vi "Drive_Execute.vi"() -> ()   [LabVIEW 2019]
uses:
  Drive_Globals.vi
  <vilib>/Rock Robotics/WPI/ThirdParty/Phoenix-LabVIEW/Motor Controller/Controls/CTRE_Phoenix_MotorControl_ControlMode.ctl
  <vilib>/Rock Robotics/WPI/Joystick/WPI_JoystickArcadeMapping.vi
panel:
  in  "Max Speed":dbl
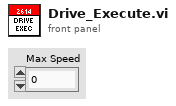
[diagram p1: front panel]
types:
  T1 = typedef "WPI_MotorControlDeviceRef.ctl" = cluster{"DeviceStatus":errorcluster, "Type":T2, "PWM":cluster{"PWM Channel":T3, "DeadBand":T4}, "CAN":cluster{"Device Number":u8, "SetOutput VI Ref":variant, "GetOutput VI Ref":variant, "Enable VI Ref":variant, "Disable VI Ref":variant, "Data":variant}, "Invert":bool, "DIO PWM":cluster{"PWM \"Enable\" Channel":T3, "DIOChannel":T5, "PWM Rate":dbl}}
  T2 = typedef "WPI_MotorControlType.ctl" = enum16{"PWM", "CAN", "DIO PWM"}
  T3 = typedef "FPGA_DIOPWMChannel.ctl" = enum8{"PWM 0", "PWM 1", "PWM 2", "PWM 3", "PWM 4", "PWM 5", "PWM 6", "PWM 7", "PWM 8", "PWM 9", "PWM MXP 0", "PWM MXP 1", "PWM MXP 2", "PWM MXP 3", "PWM MXP 4", "PWM MXP 5", "PWM MXP 6", "PWM MXP 7", "PWM MXP 8", "PWM MXP 9", "Invalid"}
  T4 = typedef "WPI_PWMDeadband.ctl" = cluster{"Name":string, "maxPositivePwm":i32, "minPositivePwm":i32, "centerPwm":i32, "maxNegativePwm":i32, "minNegativePwm":i32, "angularRange":u16}
  T5 = typedef "FPGA_DIOChannel.ctl" = enum8{"DIO 0", "DIO 1", "DIO 2", "DIO 3", "DIO 4", "DIO 5", "DIO 6", "DIO 7", "DIO 8", "DIO 9", "DIO MXP 0", "DIO MXP 1", "DIO MXP 2", "DIO MXP 3", "DIO MXP 4", "DIO MXP 5", "DIO MXP 6", "DIO MXP 7", "DIO MXP 8", "DIO MXP 9", "DIO MXP 10", "DIO MXP 11", "DIO MXP 12", "DIO MXP 13", "DIO MXP 14", "DIO MXP 15", "SPI Port CS1", "SPI Port CS2", "SPI Port CS3", "SPI Port MISO", "SPI Port MOSI", "Invalid"}
  T6 = typedef "DriveExecuteCluster.ctl" = cluster{"Front/Back":dbl, "Turn":dbl, "Drive Control Type":enum16{"PercentVoltage", "SpeedControl"}}
  T7 = typedef "CTRE_Phoenix_MotorControl_ControlMode.ctl" = u16
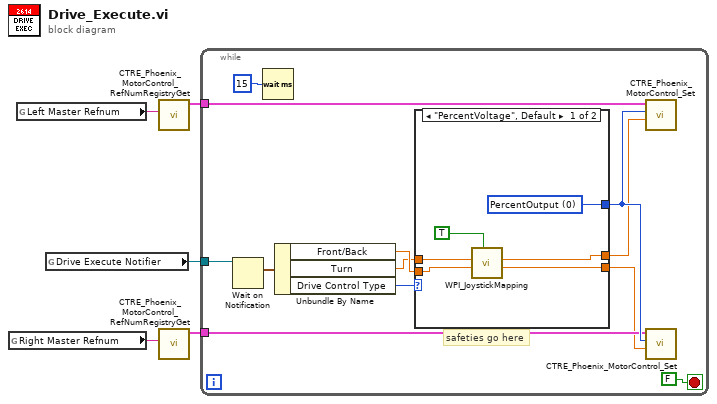
[diagram p0: block diagram]
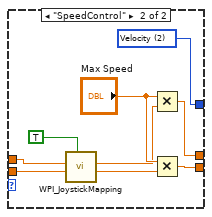
[diagram p2: hidden frame]
diagram:
  n1 = global read "Drive_Globals.vi" "Right Master Refnum"() -> (w4:string)
  n2 = global read "Drive_Globals.vi" "Left Master Refnum"() -> (w3:string)
  n3 = global read "Drive_Globals.vi" "Drive Execute Notifier"() -> (w5:refnum<notifier>)
  n4 = call <vilib>:"CTRE_Phoenix_MotorControl_RefNumRegistryGet.vi"("refnum name"=w3) -> ("PhoenixMotorControlDevRef"=w2:T1)  [unwired: 9 in, 1 out]
  n5 = call <vilib>:"CTRE_Phoenix_MotorControl_RefNumRegistryGet.vi"("refnum name"=w4) -> ("PhoenixMotorControlDevRef"=w1:T1)  [unwired: 9 in, 1 out]
  n6 = while {
    tunnel: w5 -> [w15]
    tunnel: w2 -> [w9]
    tunnel: w1 -> [w8]
    stop <- FALSE stop-if-true
    # "safeties go here"
    n7 = Wait on Notification(notifier=w15) -> (notification=w14:T6)  [unwired: 3 in, 3 out]
    n8 = Wait (ms)(milliseconds to wait=u32 15) -> ()  [unwired: 1 out]
    n9 = Unbundle By Name(w14) -> ("Front/Back"=w11:dbl, "Turn"=w10:dbl, "Drive Control Type"=w13:enum16{"PercentVoltage", "SpeedControl"})
    n10 = case shown="\"PercentVoltage\", Default" w13 {
      tunnel: [w23 w32] -> w12
      tunnel: w11 -> [w22 w31]
      tunnel: w10 -> [w21 w30]
      tunnel: [w20 w28] -> w7
      tunnel: [w19 w24] -> w6
      frame "PercentVoltage", Default {
        w23 = T7 0 items=["PercentOutput"=0, "Position"=1, "Velocity"=2, "Current"=3, "Follower"=5, "MotionProfile"=6, "MotionMagic"=7, "MotionProfileArc"=10, "Disabled"=15] ("Control Mode")
        n11 = call-poly <vilib>:"WPI_JoystickMapping.vi"("Square Inputs"=TRUE, "Y axis value"=w22, "X axis value"=w21) -> ("Right Motor Value"=w19:dbl, "Left Motor Value"=w20:dbl)  [unwired: 7 in]
      }
      frame "SpeedControl" {
        w32 = T7 2 items=["PercentOutput"=0, "Position"=1, "Velocity"=2, "Current"=3, "Follower"=5, "MotionProfile"=6, "MotionMagic"=7, "MotionProfileArc"=10, "Disabled"=15] ("Control Mode")
        n12 = call-poly <vilib>:"WPI_JoystickMapping.vi"("Square Inputs"=TRUE, "Y axis value"=w31, "X axis value"=w30) -> ("Right Motor Value"=w25:dbl, "Left Motor Value"=w26:dbl)  [unwired: 7 in]
        n13 = Multiply(x="Max Speed", y=w26) -> (x*y=w28:dbl)
        n14 = Multiply(x="Max Speed", y=w25) -> (x*y=w24:dbl)
      }
    }
    n15 = call <vilib>:"CTRE_Phoenix_MotorControl_Set.vi"("Output"=w7, "Control Mode"=w12, "PhoenixMotorControlDevRef"=w9) -> ()  [unwired: 7 in, 2 out]
    n16 = call <vilib>:"CTRE_Phoenix_MotorControl_Set.vi"("Output"=w6, "Control Mode"=w12, "PhoenixMotorControlDevRef"=w8) -> ()  [unwired: 7 in, 2 out]
  }
